vi "XRange.vi"(0 "SygZad Podg Ref":refnum<vi>, 1 "Radio Buttons":T1(radio), 2 "Offset DistAC":dbl, 3 "Amplituda":dbl, 4 "Offset":dbl, 5 "error in (no error)":errorcluster) -> (19 "error out":errorcluster)   [LabVIEW 2021]
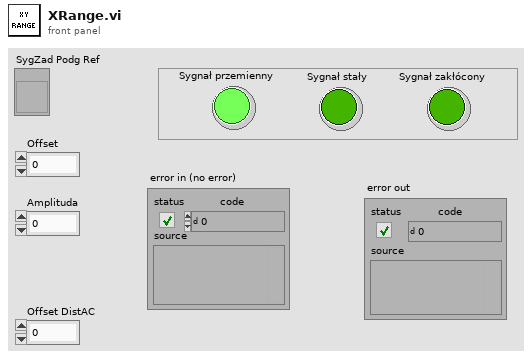
[diagram p1: front panel]
types:
  T1 = enum32{"Sygnał przemienny", "Sygnał stały", "Sygnał zakłócony"}
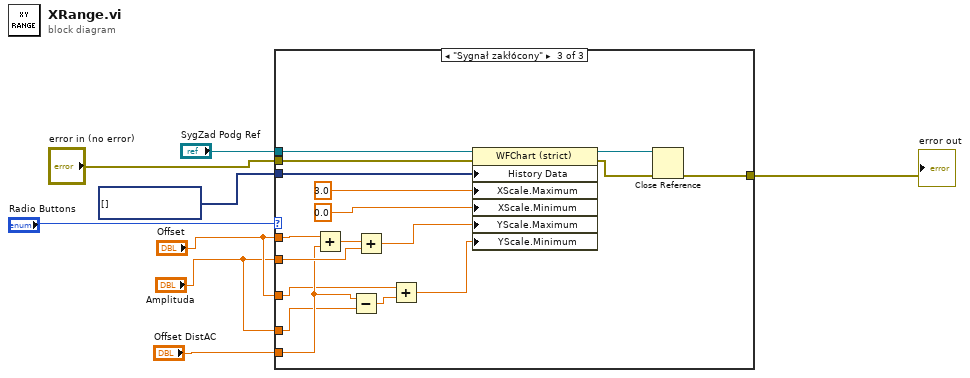
[diagram p0: block diagram]
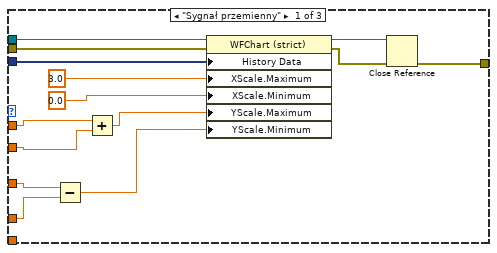
[diagram p2: hidden frame]
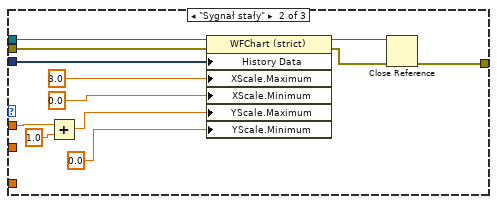
[diagram p3: hidden frame]
diagram:
  n1 = case shown="\"Sygnał zakłócony\"" "Radio Buttons" {
    tunnel: "SygZad Podg Ref" -> [w22 w34 w51]
    tunnel: "error in (no error)" -> [w20 w32 w49]
    tunnel: [w18 w30 w47] -> w6
    tunnel: dynamicdata[] [] ("History Data") -> [w17 w29 w46]
    tunnel: "Offset" -> [w9 w26 w43]
    tunnel: "Amplituda" -> [w13 _ w41]
    tunnel: "Offset" -> [w12 _ w36]
    tunnel: "Amplituda" -> [w11 _ w38]
    tunnel: "Offset DistAC" -> [_ _ w39]
    frame "Sygnał przemienny" {
      n2 = Subtract(x=w12, y=w11) -> (x-y=w10:dbl)
      n3 = Add(x=w9, y=w13) -> (x+y=w14:dbl)
      n4 = property class="WFChart (strict)"(reference=w22, error in=w20, "History Data"=w17, "XScale.Maximum"=3.0 ("X Scale.Range:Maximum"), "XScale.Minimum"=0.0 ("X Scale.Range:Minimum"), "YScale.Maximum"=w14, "YScale.Minimum"=w10) -> (reference out=w21:refnum<vi>, error out=w19:errorcluster)
      n5 = Close Reference(reference=w21, error in (no error)=w19) -> (error out=w18:errorcluster)
    }
    frame "Sygnał stały" {
      n6 = Add(x=w26, y=1.0) -> (x+y=w25:dbl)
      n7 = property class="WFChart (strict)"(reference=w34, error in=w32, "History Data"=w29, "XScale.Maximum"=3.0 ("X Scale.Range:Maximum"), "XScale.Minimum"=0.0 ("X Scale.Range:Minimum"), "YScale.Maximum"=w25, "YScale.Minimum"=0.0 ("Y Scale.Range:Minimum")) -> (reference out=w33:refnum<vi>, error out=w31:errorcluster)
      n8 = Close Reference(reference=w33, error in (no error)=w31) -> (error out=w30:errorcluster)
    }
    frame "Sygnał zakłócony" {
      n9 = Add(x=w43, y=w39) -> (x+y=w42:dbl)
      n10 = Subtract(x=w39, y=w38) -> (x-y=w37:dbl)
      n11 = Add(x=w42, y=w41) -> (x+y=w40:dbl)
      n12 = Add(x=w36, y=w37) -> (x+y=w35:dbl)
      n13 = property class="WFChart (strict)"(reference=w51, error in=w49, "History Data"=w46, "XScale.Maximum"=3.0 ("X Scale.Range:Maximum"), "XScale.Minimum"=0.0 ("X Scale.Range:Minimum"), "YScale.Maximum"=w40, "YScale.Minimum"=w35) -> (reference out=w50:refnum<vi>, error out=w48:errorcluster)
      n14 = Close Reference(reference=w50, error in (no error)=w48) -> (error out=w47:errorcluster)
    }
  }
  "error out" <- w6
